vi "RD Analog In Status.vi"(8 "error in (no error)":errorcluster caption="错误输入（无错误）", 11 "handle":u64) -> (0 "error out":errorcluster caption="错误输出", 1 "function return":i32, 2 "ANIStatus":T1(ring), 3 "handle out":u64)   [LabVIEW 2018, in "InstrumentsPlayground.lvlib"]
doc: "CLIFFAPI int CliffAnalogInStatus(FT_HANDLE handle,CLIFFState* sts);\nconst CLIFFState CLIFFStateReady = 0;\nconst CLIFFState CLIFFStateConfig = 4;\nconst CLIFFState CLIFFStatePrefill = 5;\nconst CLIFFState CLIFFStateArmed = 1;\nconst CLIFFState CLIFFStateWait = 7;\nconst CLIFFState CLIFFStateTriggered = 3;\nconst CLIFFState CLIFFStateRunning = 3;\nconst CLIFFState CLIFFStateDone = 2;"
uses:
  InstrumentsPlayground.lvlib
panel:
  out "sts out":string
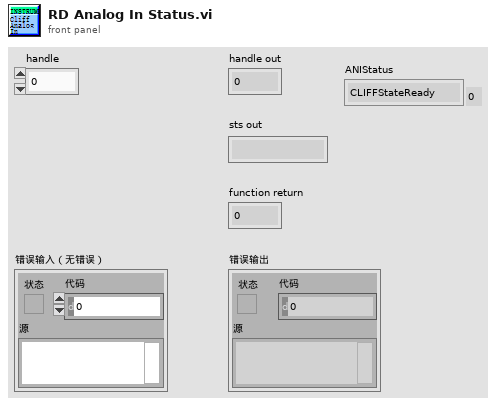
[diagram p1: front panel]
types:
  T1 = enum16{"CLIFFStateReady", "CLIFFStateArmed", "CLIFFStateDone", "CLIFFStateRunning", "CLIFFStateConfig", "CLIFFStatePrefill", "CLIFFStateTriggered", "CLIFFStateWait"}
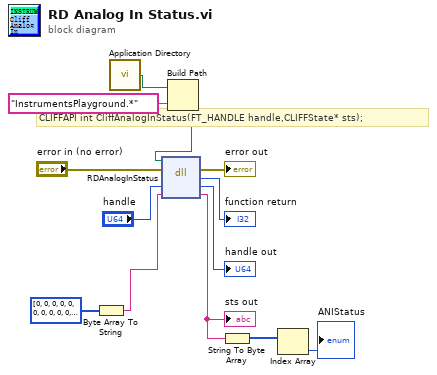
[diagram p0: block diagram]
diagram:
  # "CLIFFAPI int CliffAnalogInStatus(FT_HANDLE handle,CLIFFState* sts);"
  n1 = Byte Array To String(unsigned byte array=u8[] [0, 0, 0, 0, 0, 0, 0, 0, 0, 0, 0] ("无符号字节数组")) -> (string=w5:string)
  n2 = call <vilib>:"Application Directory.vi"() -> ("Application Directory"=w2:path)
  n3 = Build Path(base path=w2, name or relative path="InstrumentsPlayground.*" ("名称或相对路径")) -> (appended path=w1:path)
  n4 = dll-call lib="E:/work/YZCourse_Xtext/Cliff/API/LabVIEW lib/InstrumentsPlayground.*" fn="RDAnalogInStatus"(path in=w1, error in="error in (no error)", "handle"="handle", "sts"=w5) -> (error out=→"error out":errorcluster, "返回类型"=→"function return":i32, "handle"=→"handle out":u64, "sts"=w8:string)  [unwired: 1 in, 1 out]
  "sts out" <- w8
  n5 = String To Byte Array(string=w8) -> (unsigned byte array=w7:u8[])
  n6 = Index Array(array=w7) -> (element=→"ANIStatus":u8)  [unwired: 1 in]
